vi "init.vi"() -> (0 "man mode":bool, 1 "Array":i32[][](array[numeric])=[[0, 2, 3, 2, 1], [1, 0, 0, 3, 1], [2, 1, 3, 3, 1], [3, 3, 1, 2, 1], [4, 5, 0, 3, 1], [5, 1, 0, 2, 2], [6, 3, 0, 2, 2], [7, 1, 2, 2, 2], [8, 3, 3, 3, 2], [9, 4, 4, 2, 2], [10, 2, 5, 2, 2], [11, 4, 5, 2, 2]], 2 "element":string)   [LabVIEW 2021]
panel:
  out "computer mode":bool
  in  "Boolean":bool
  in  "stop":bool
  in  "Ring":u16(ring) items=["very easy", "easy", "medium", "hard", "very hard"]
  out "all rows":i64[][](array[numeric])
  out "32bit integer":i32
  out "size(s)":i32
  out "filenames":string[](array[string])
  out "appended path":path
  out "Ready":bool
  # "Choose difficulty you want"
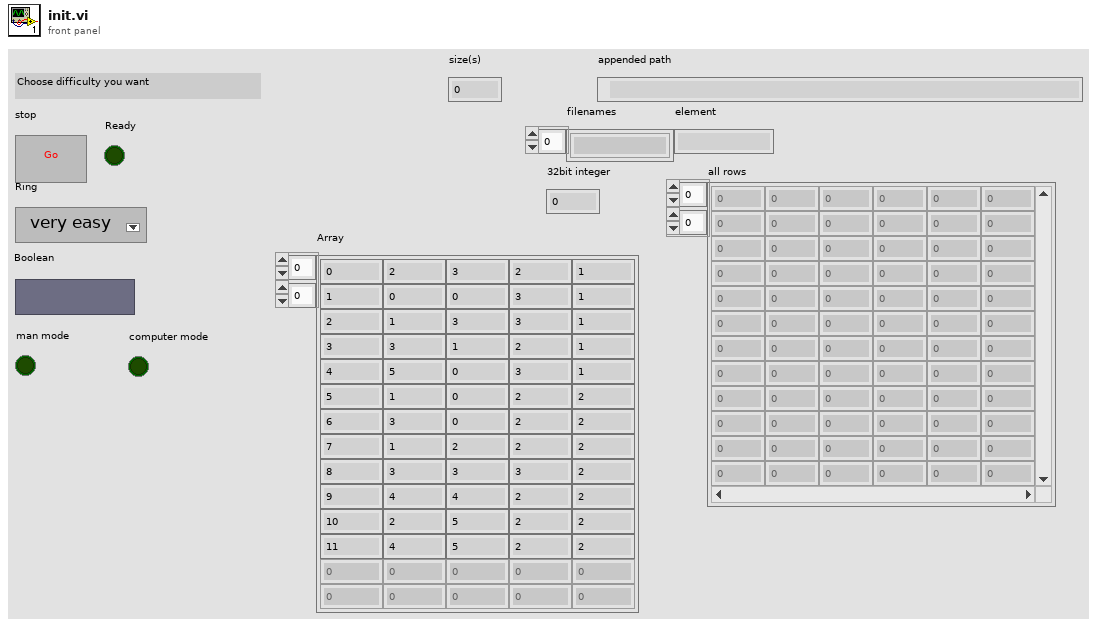
[diagram p1: front panel]
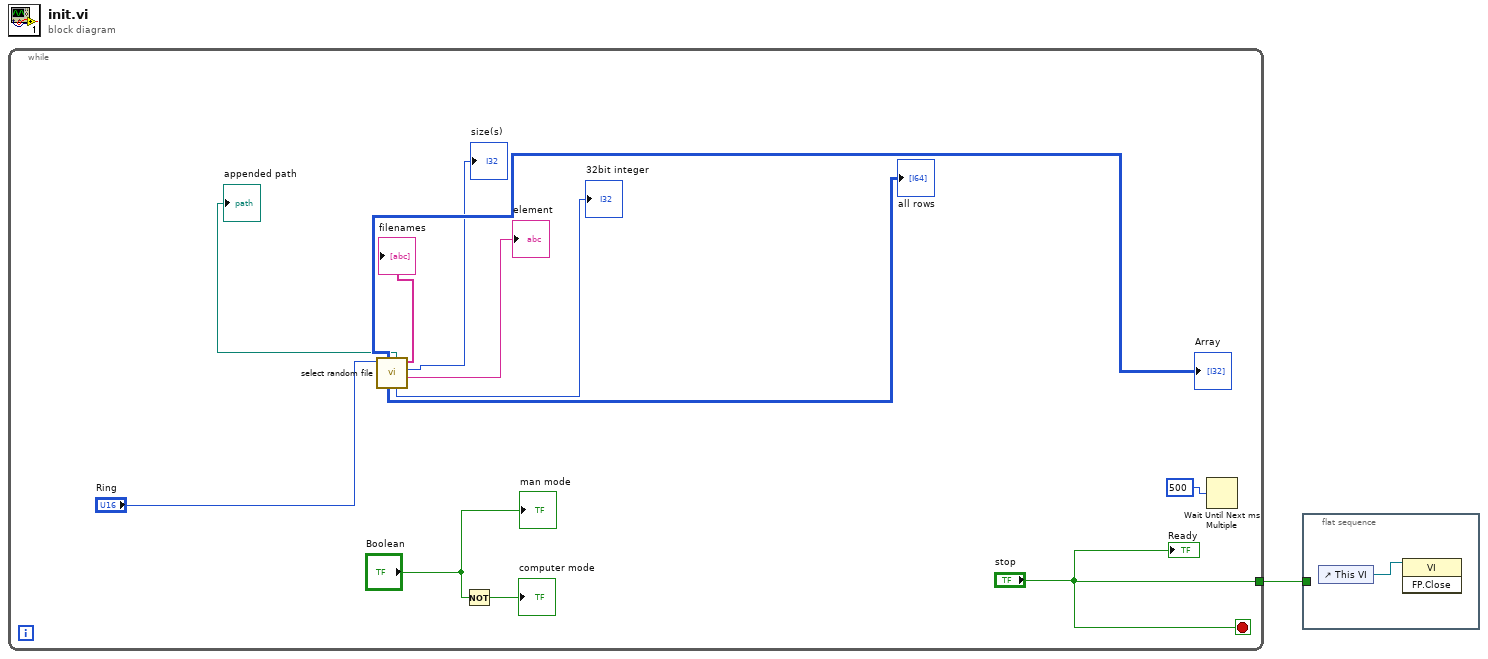
[diagram p0: block diagram]
diagram:
  n1 = while {
    tunnel: ["stop"] -> w1
    stop <- "stop" stop-if-true
    n2 = call "select random file.vi"("Ring"="Ring") -> ("element"=→"element":string, "size(s)"=→"size(s)":i32, "filenames"=→"filenames":string[], "32bit integer"=→"32bit integer":i32, "appended path"=→"appended path":path, "all rows"=→"all rows":i64[][], "all rows 2"=→"Array":i64[][])  [unwired: 4 in]
    n3 = Not(x="Boolean") -> (.not. x?=→"computer mode":bool)
    n4 = Wait Until Next ms Multiple(millisecond multiple=u32 500) -> ()  [unwired: 1 out]
    "Ready" <- "stop"
    "man mode" <- "Boolean"
  }
  n5 = flat-sequence {
    tunnel: w1 -> [_]
    frame #0 {
      n6 = control-ref of="This VI"() -> (w14:refnum<vi>)
      n7 = invoke class="VI" method="FP.Close"(reference=w14) -> ()  [unwired: 2 in, 3 out]
    }
  }
